vi "crest.vi"(6 "Set / Unit?":enum16{"Unit", "SetUp"}(ring), 8 "Error In":errorcluster, 9 "SetUP W":T1(ring), 10 "SetUP F":dbl, 11 "RMS":dbl) -> (0 "Error Out":errorcluster, 3 "Max":dbl)   [LabVIEW 2021, in "Signal.lvlib"]
doc: "This subvi is used to calculate the max value of the signal."
uses:
  Signal.lvlib
  Tipski Definicii/Signal Values.ctl
panel:
  # "Output"
  # "Input"
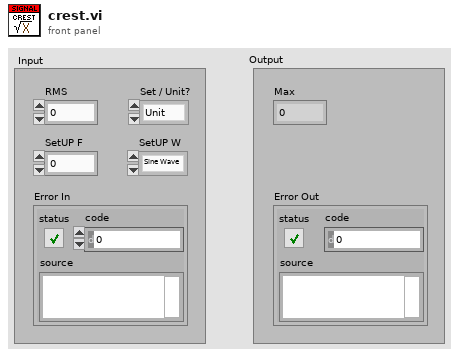
[diagram p1: front panel]
types:
  T1 = enum16{"Sine Wave", "Triangle Wave", "Square Wave", "Sawtooth Wave"}
  T2 = typedef "Signal Values.ctl" = enum16{"Init", "Add V/A string", "Add Hz string", "Get Strings and Values", "Reset", "Add Offset", "Add Waveform", "Add Phase"}
  T3 = cluster{"Amp String":string, "Amp Value":dbl, "Hz Value Out":dbl, "Waveform Out":enum16{"Sine Wave", "Triangle Wave", "Square Wave", "Sawtooth Wave"}, "Offset Out":dbl, "Phase Out":dbl, "Signal String":string, "Signal":waveform(dbl)}
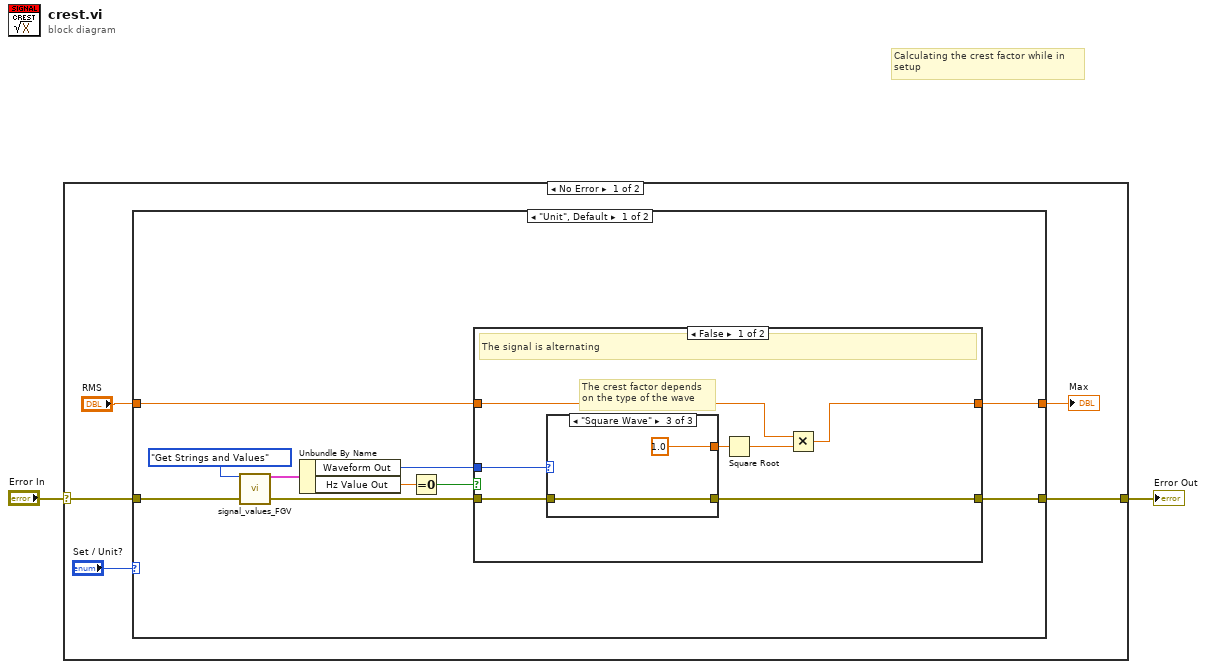
[diagram p0: block diagram]
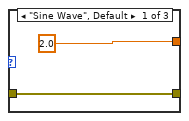
[diagram p2: hidden frame]
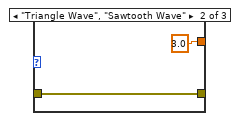
[diagram p3: hidden frame]
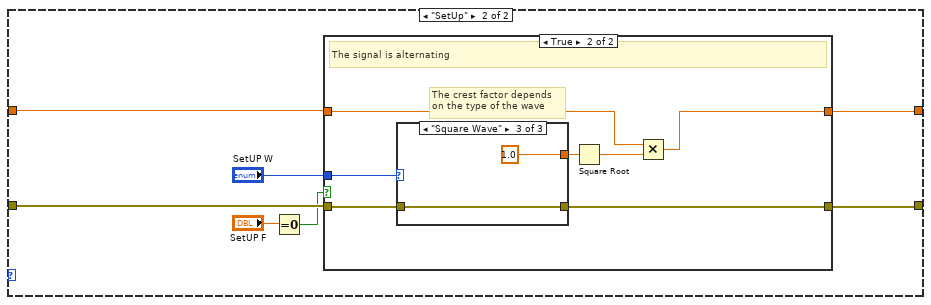
[diagram p5: hidden frame]
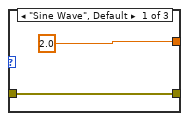
[diagram p7: hidden frame]
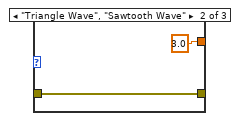
[diagram p8: hidden frame]
diagram:
  # "Calculating the crest factor while in \nsetup"
  n1 = case shown="No Error" "Error In" {
    selector: "Error In" -> [w7 w55]
    tunnel: [w6 w55] -> w1
    frame No Error {
      n2 = case shown="\"Unit\", Default" "Set / Unit?" {
        tunnel: w7 -> [w16 w39]
        tunnel: [w11 w34] -> w6
        tunnel: "RMS" -> [w10 w37]
        tunnel: [w9 w33] -> w3
        frame "Unit", Default {
          n3 = call "signal_values_FGV.vi"("Action"=Signal_Values."Get Strings and Values", "Error In"=w16) -> ("Signal"=w15:T3, "Error Out"=w13:errorcluster)  [unwired: 12 in]
          n4 = Unbundle By Name(w15) -> ("Waveform Out"=w14:T1, "Hz Value Out"=w12:dbl)
          n5 = Equal To 0?(x=w12) -> (x = 0?=w8:bool)
          n6 = case shown="False" w8 {
            tunnel: w14 -> [w24 _]
            tunnel: w13 -> [w23 w31]
            tunnel: w10 -> [w21 w32]
            tunnel: [w19 w32] -> w9
            tunnel: [w18 w31] -> w11
            frame False {
              # "The crest factor depends \non the type of the wave"
              # "The signal is alternating"
              n7 = case shown="\"Square Wave\"" w24 {
                tunnel: [2.0 3.0 1.0] -> w20
                tunnel: w23 -> [w25 w27 w29]
                tunnel: [w25 w27 w29] -> w18
                frame "Sine Wave", Default {
                }
                frame "Triangle Wave", "Sawtooth Wave" {
                }
                frame "Square Wave" {
                }
              }
              n8 = Square Root(x=w20) -> (sqrt(x)=w22:dbl)
              n9 = Multiply(x=w21, y=w22) -> (x*y=w19:dbl)
            }
            frame True {
              # "The signal is direct"
            }
          }
        }
        frame "SetUp" {
          n10 = Equal To 0?(x="SetUP F") -> (x = 0?=w35:bool)
          n11 = case shown="True" w35 {
            tunnel: "SetUP W" -> [_ w48]
            tunnel: w39 -> [w40 w47]
            tunnel: w37 -> [w41 w45]
            tunnel: [w41 w43] -> w33
            tunnel: [w40 w42] -> w34
            frame False {
              # "The signal is direct"
            }
            frame True {
              # "The crest factor depends \non the type of the wave"
              # "The signal is alternating"
              n12 = case shown="\"Square Wave\"" w48 {
                tunnel: [2.0 3.0 1.0] -> w44
                tunnel: w47 -> [w49 w51 w53]
                tunnel: [w49 w51 w53] -> w42
                frame "Sine Wave", Default {
                }
                frame "Triangle Wave", "Sawtooth Wave" {
                }
                frame "Square Wave" {
                }
              }
              n13 = Square Root(x=w44) -> (sqrt(x)=w46:dbl)
              n14 = Multiply(x=w45, y=w46) -> (x*y=w43:dbl)
            }
          }
        }
      }
      "Max" <- w3
    }
    frame Error {
    }
  }
  "Error Out" <- w1
